vi "nanocal -- nuclear schottky fit V5.vi"() -> ()   [LabVIEW 2020] (continued)
                n371 = Or(x=w756, y=w763) -> (x .or. y?=w767:bool)
              }
              n372 = And Array Elements(Boolean array=w753) -> (logical AND=w752:bool)
            }
            n373 = for {
              tunnel: [w785] -> w748 mode=indexing
              tunnel: [w783] -> w746 mode=indexing
              tunnel: [w780] -> w750 mode=indexing
              tunnel: w744 -> [w782] mode=indexing
              tunnel: w740 -> [w781]
              n374 = Unbundle(w782) -> ("event data"=w780:string, "file pattern"=w785:string)
              n375 = local read "X selector"() -> (w779:T1)
              n376 = Look In Map(map=w781, key=w780) -> (value=w784:map{T1, dbl})  [unwired: 1 in, 1 out]
              n377 = Look In Map(map=w784, key=w779) -> (value=w783:dbl)  [unwired: 1 in, 1 out]
            }
            n378 = call "array - sorted inexes.vi"("x"=w746) -> ("index array"=w747:i32[])  [unwired: 9 in, 1 out]
            n379 = for {
              tunnel: w747 -> [w775] mode=indexing
              tunnel: w748 -> [w778]
              tunnel: [w777] -> w749 mode=indexing
              tunnel: w750 -> [w776]
              shift-right: [w771] -> w739
              shift-left: w745 -> [w774]
              i -> [w773]
              n380 = Index Array(array=w778, index=w775) -> (element=w777:string)
              n381 = Index Array(array=w776, index=w775) -> (element=w772:string)
              n382 = Insert Into Map(map in=w774, key=w773, value=w772) -> (map out=w771:map{i32, string})  [unwired: 2 out]
            }
            "constrained filename lookup" <- w739
            n383 = property on="selection :|\\" class="Ring (strict)"("Strings []"=w749) -> ()  [unwired: 2 in, 2 out]
          }
          frame "action: constrained filenames select" {
            n384 = local read "constrained filename lookup"() -> (w788:map{i32, string})
            n385 = local read "selection :|\\"() -> (w789:u16)
            n386 = local read "all full filenames"() -> (w790:map{string, path})
            n387 = Look In Map(map=w788, key=w789) -> (value=w791:string)  [unwired: 1 in, 1 out]
            n388 = Look In Map(map=w790, key=w791) -> (value=w792:path)  [unwired: 1 in, 1 out]
            n389 = for {
              N: 1 -> [_]
              tunnel: w786 -> [w794]
              tunnel: w792 -> [w793]
              n390 = local write "Read from file"(w793) -> ()
              n391 = Generate User Event(user event=w794, event data cluster="action: read from file" ("event data")) -> ()  [unwired: 2 in, 2 out]
            }
          }
          frame "action: write mathematica string" {
            n392 = local read "mathematica thing"() -> (w800:map{string, map{T1, dbl}})
            n393 = local read "folder"() -> (w799:path)
            n394 = Build Path(base path=w799, name or relative path="temporarystring.txt") -> (appended path=w798:path)
            n395 = call "string parse mathematica list assosiated array -- V2.vi"("action"=3-lorentzian-heat-response_action."create string" ("derivative"), "Map IN"=w800) -> ("string out"=w796:string)  [unwired: 8 in, 1 out]
            "string OUT" <- w796
            n396 = Write to Text File(file (use dialog)=w798, text=w796) -> ()  [unwired: 2 in, 3 out]
          }
          frame "action: replot colors" {
            # "all -- including kappa0"
            n397 = local read "new selector names"() -> (w811:map{T1, map{T10, string}})
            n398 = local read "state of all selectors"() -> (w829:map{T1, map{bool, dbl}})
            n399 = local read "mathematica thing"() -> (w834:map{string, map{T1, dbl}})
            n400 = local read "X selector"() -> (w804:T1)
            n401 = case shown="\"B (T)\"" w804 {
              tunnel: ["B (T)" "T (K)"] -> w803
              frame "B (T)" {
              }
              frame "T (K)", Default {
              }
            }
            n402 = Look In Map(map=w811, key=w804) -> (value=w810:map{T10, string})  [unwired: 1 in, 1 out]
            n403 = control-ref of="Plot:  colors"() -> (w806:refnum<vi>)
            n404 = Array Subset(array=w833, index=0, length=6 ("index")) -> (w831:T1[])
            n405 = local read "state of all selectors string"() -> (w802:string)
            n406 = Look In Map(map=w810, key=nameformattingitem."nameL") -> (value=w808:string)  [unwired: 1 in, 1 out]
            n407 = call "replace plot - plot ref - V2.vi"("Plot ref in"=w806, "text"=w803, "cursor action"=cursor_action."set Xlabel") -> ("Plot ref out"=w805:refnum<vi>)  [unwired: 13 in, 3 out]
            n408 = Concatenate Strings(w802, w808) -> (w828:string)
            n409 = for {
              tunnel: w834 -> [w873]
              tunnel: w804 -> [w868]
              tunnel: w831 -> [w856] mode=indexing
              tunnel: w829 -> [w869]
              tunnel: w811 -> [w860]
              shift-right: [w864] -> w820
              shift-left: w828 -> [w867]
              tunnel: w802 -> [w865]
              tunnel: [w861] -> w822 mode=indexing
              tunnel: w805 -> [w853]
              n410 = for {
                tunnel: w873 -> [w900] mode=indexing
                tunnel: w856 -> [w899]
                tunnel: [w898] -> w872 mode=indexing if=w892
                tunnel: [w897] -> w871 mode=indexing if=w892
                tunnel: w868 -> [w896]
                tunnel: w869 -> [w895]
                n411 = Unbundle(w900) -> ("Map"=w894:map{T1, dbl})  [unwired: 1 out]
                n412 = for {
                  tunnel: w895 -> [w909] mode=indexing
                  tunnel: w894 -> [w908]
                  tunnel: [w906] -> w893 mode=indexing
                  n413 = Unbundle(w909) -> ("Plost: sweep window"=w907:T1, "map"=w905:map{bool, dbl})
                  n414 = for {
                    tunnel: w905 -> [w912] mode=indexing
                    tunnel: [w911] -> w902
                    tunnel: [w910] -> w903
                    n415 = Unbundle(w912) -> ("ignore side !"=w911:bool, "number OUT"=w910:dbl)
                  }
                  n416 = Look In Map(map=w908, key=w907) -> (value=w904:dbl)  [unwired: 1 in, 1 out]
                  n417 = Equal?(x=w904, y=w903) -> (x = y?=w901:bool)
                  n418 = Or(x=w902, y=w901) -> (x .or. y?=w906:bool)
                }
                n419 = Look In Map(map=w894, key=w896) -> (value=w898:dbl)  [unwired: 1 in, 1 out]
                n420 = Look In Map(map=w894, key=w899) -> (value=w897:dbl)  [unwired: 1 in, 1 out]
                n421 = And Array Elements(Boolean array=w893) -> (logical AND=w892:bool)
              }
              n422 = Look In Map(map=w860, key=w856) -> (value=w858:map{T10, string})  [unwired: 1 in, 1 out]
              n423 = Look In Map(map=w858, key=nameformattingitem."nameL") -> (value=w857:string)  [unwired: 1 in, 1 out]
              n424 = call <vilib>:"Space Constant.vi"() -> ("String"=w866:string)
              n425 = Concatenate Strings(w867, w866, w865, w857) -> (w864:string)
              n426 = local read "cursor index map"() -> (w854:map{T1, i32})
              n427 = call "array - sorted inexes.vi"("x"=w872) -> ("index array"=w870:i32[])  [unwired: 9 in, 1 out]
              n428 = local read "color Map"() -> (w855:map{T1, u32})
              n429 = for {
                tunnel: w872 -> [w891]
                tunnel: w871 -> [w890]
                tunnel: w870 -> [w887] mode=indexing
                tunnel: [w889] -> w863 mode=indexing
                tunnel: [w888] -> w862 mode=indexing
                n430 = Index Array(array=w891, index=w887) -> (element=w889:dbl)
                n431 = Index Array(array=w890, index=w887) -> (element=w888:dbl)
              }
              n432 = case shown="\"ζ\"..\"τC\", Default" w856 {
                selector: w856 -> [_ w882]
                tunnel: w863 -> [_ w884]
                tunnel: w862 -> [_ w883]
                tunnel: w855 -> [_ w881]
                tunnel: w854 -> [_ w880]
                tunnel: w853 -> [_ w879]
                frame "κ0" {
                }
                frame "ζ".."τC", Default {
                  n433 = Look In Map(map=w880, key=w882) -> (value=w875:i32)  [unwired: 1 in, 1 out]
                  n434 = call "replace plot - plot ref - V2.vi"("Plot ref in"=w879, "Array X IN"=w884, "Array Y IN"=w883, "plot index"=w875, "cursor action"=cursor_action."write") -> ("Plot ref out"=w878:refnum<vi>)  [unwired: 11 in, 3 out]
                  n435 = Look In Map(map=w881, key=w882) -> (value=w874:u32)  [unwired: 1 in, 1 out]
                  n436 = call "replace cursor - plot ref - V2.vi"("Plot ref in"=w878, "cursor index"=w875, "cursor action"=cursor_action."set cursor color", "Color Box"=w874) -> ("Plot ref out"=w877:refnum<vi>)  [unwired: 12 in, 3 out]
                  n437 = call "replace plot - plot ref - V2.vi"("Plot ref in"=w877, "plot index"=w875, "cursor action"=cursor_action."set plot color", "Color Box"=w874) -> ()  [unwired: 12 in, 4 out]
                }
              }
              n438 = Bundle(w863, w862) -> (w861:cluster{dbl[], dbl[]})  [unwired: 1 in]
            }
            n439 = Index Array(array=w822, index=0) -> (element=w826:cluster{dbl[], dbl[]})
            n440 = local read "folder"() -> (w817:path)
            n441 = Unbundle(w826) -> (w825:dbl[])  [unwired: 1 out]
            n442 = Concatenate Strings("plotstring", w802, ".dat") -> (w812:string)
            n443 = Concatenate Strings(w820, "\r") -> (w818:string)
            n444 = Build Array(w825) -> (w824:dbl[][])
            n445 = for {
              shift-right: [w850] -> w823
              shift-left: w824 -> [w852]
              tunnel: w822 -> [w849] mode=indexing
              n446 = Unbundle(w849) -> (w851:dbl[])  [unwired: 1 out]
              n447 = Build Array (concatenate)(w852, w851) -> (w850:dbl[][])
            }
            n448 = Build Path(base path=w817, name or relative path=w812) -> (appended path=w816:path)
            n449 = Transpose 2D Array(2D array=w823) -> (transposed array=w821:dbl[][])
            n450 = for {
              shift-right: [w842] -> w815
              shift-left: w818 -> [w841]
              tunnel: w821 -> [w839] mode=indexing
              n451 = for {
                shift-right: [w843] -> w838
                shift-left: "" -> [w848]
                tunnel: w839 -> [w847] mode=indexing
                n452 = Number To Fractional String(number=w847, precision (6)=i16 16) -> (F-format string=w845:string)  [unwired: 2 in]
                n453 = Concatenate Strings(w848, w845, "    ") -> (w843:string)
              }
              n454 = Concatenate Strings(w841, w838, "\r") -> (w842:string)
            }
            n455 = Write to Text File(file (use dialog)=w816, text=w815) -> ()  [unwired: 2 in, 3 out]
          }
          frame "action: update state of selectors" {
            w932 = T1[] [enum."T (K)", enum."B (T)", enum."θ (deg)", enum."side (S|R)"] items=["ζ", "τ1", "τS", "τN", "τC", "κ0", "m1", "m2", "m3", "T (K)", "B (T)", "θ (deg)", "side (S|R)", "set of (B|T)", "Re(offset)", "Im(offset)"]
            n456 = local read "selector"() -> (w928:T12)
            n457 = local read "new selector names"() -> (w935:map{T1, map{T10, string}})
            n458 = Unbundle By Name(w928) -> ("side (8S|4R)"=w927:i32, "ignore side !"=w926:bool, "lookup.side lookup"=w925:map{i32, dbl}, "T (K)"=w922:u16, "ignore T !"=w924:bool, "lookup.T lookup"=w923:map{i32, dbl}, "B (T)"=w919:u16, "ignore B !"=w921:bool, "lookup.B lookup"=w920:map{i32, dbl}, "θ (deg)"=w917:u16, "ignore θ !"=w916:bool, "lookup.θ lookup"=w918:map{i32, dbl}, "set (1T|2B)"=w913:i32, "ignore set of !"=w914:bool, "lookup.set of lookup"=w915:map{i32, dbl})
            n459 = Generate User Event(user event=w937, event data cluster="action: replot colors" ("event data")) -> (user event out=w938:refnum<user-event>)  [unwired: 2 in, 1 out]
            n460 = Generate User Event(user event=w938, event data cluster="action: update constrained file selector" ("event data")) -> ()  [unwired: 2 in, 2 out]
            n461 = Look In Map(map=w925, key=w927) -> (value=w931:dbl)  [unwired: 1 in, 1 out]
            n462 = node(w926, w931) -> (w953:map{bool, dbl})
            n463 = Look In Map(map=w923, key=w922) -> (value=w952:dbl)  [unwired: 1 in, 1 out]
            n464 = Look In Map(map=w920, key=w919) -> (value=w948:dbl)  [unwired: 1 in, 1 out]
            n465 = node(w924, w952) -> (w950:map{bool, dbl})
            n466 = node(w921, w948) -> (w947:map{bool, dbl})
            n467 = Look In Map(map=w918, key=w917) -> (value=w946:dbl)  [unwired: 1 in, 1 out]
            n468 = node(w916, w946) -> (w944:map{bool, dbl})
            n469 = Look In Map(map=w915, key=w913) -> (value=w943:dbl)  [unwired: 1 in, 1 out]
            n470 = node(w914, w943) -> (w941:map{bool, dbl})
            n471 = local read "side map from NUM"() -> (w929:map{i32, T8})
            n472 = node(3-lorentzian-parameters."side (S|R)" ("Plost: sweep window"), w953, 3-lorentzian-parameters."T (K)" ("Plost: sweep window"), w950, 3-lorentzian-parameters."B (T)" ("Plost: sweep window"), w947, 3-lorentzian-parameters."θ (deg)" ("Plost: sweep window"), w944, 3-lorentzian-parameters."set of (B|T)" ("Plost: sweep window"), w941) -> (w936:map{T1, map{bool, dbl}})
            "state of all selectors" <- w936
            n473 = for {
              shift-right: [w961] -> _
              shift-left: w936 -> [w961]
              tunnel: w935 -> [w957]
              shift-right: [w960] -> w933
              shift-left: "_" ("event data") -> [w959]
              tunnel: w932 -> [w956] mode=indexing
              n474 = Look In Map(map=w957, key=w956) -> (value=w955:map{T10, string})  [unwired: 1 in, 1 out]
              n475 = Look In Map(map=w961, key=w956) -> (value=w963:map{bool, dbl})  [unwired: 1 in, 1 out]
              n476 = for {
                tunnel: w963 -> [w978] mode=indexing
                tunnel: [w977] -> w962
                tunnel: [w976] -> w958
                n477 = Unbundle(w978) -> ("ignore side ! 2"=w977:bool, "number OUT"=w976:dbl)
              }
              n478 = case shown="False" w962 {
                tunnel: [w974 w975] -> w960
                tunnel: w959 -> [w973 w975]
                tunnel: w958 -> [w970 _]
                tunnel: w955 -> [w966 _]
                frame False {
                  n479 = Look In Map(map=w966, key=nameformattingitem."prec") -> (value=w964:string)  [unwired: 1 in, 1 out]
                  n480 = Look In Map(map=w966, key=nameformattingitem."units") -> (value=w967:string)  [unwired: 1 in, 1 out]
                  n481 = Format Value(format string=w964, value (0)=w970) -> (output string=w969:string)  [unwired: 1 in]
                  n482 = Concatenate Strings(w973, "_" ("event data"), w969, w967, "_" ("event data")) -> (w974:string)
                }
                frame True {
                }
              }
            }
            "state of all selectors string" <- w933
            n483 = Look In Map(map=w929, key=w931) -> (value=w930:T8)  [unwired: 1 in, 1 out]
            n484 = local write "side"(w930) -> ()
          }
          frame "action: reset colors" {
            w985 = map{T1, u32} {}  # Size: 0
            n485 = local read "parameter"() -> (w992:T1[])
            n486 = local read "colors"() -> (w994:u32[])
            n487 = for {
              shift-right: [w997] -> w993
              shift-left: w985 -> [w998]
              tunnel: w992 -> [w996] mode=indexing
              tunnel: w994 -> [w995] mode=indexing
              n488 = Insert Into Map(map in=w998, key=w996, value=w995) -> (map out=w997:map{T1, u32})  [unwired: 2 out]
            }
            n489 = local write "color Map"(w993) -> ()
            n490 = Look In Map(map=w993, key=3-lorentzian-parameters."ζ" ("Plost: sweep window")) -> (value=w991:u32)  [unwired: 1 in, 1 out]
            n491 = Look In Map(map=w993, key=3-lorentzian-parameters."τ1" ("Plost: sweep window")) -> (value=w990:u32)  [unwired: 1 in, 1 out]
            n492 = Look In Map(map=w993, key=3-lorentzian-parameters."τS" ("Plost: sweep window")) -> (value=w989:u32)  [unwired: 1 in, 1 out]
            n493 = Look In Map(map=w993, key=3-lorentzian-parameters."τN" ("Plost: sweep window")) -> (value=w988:u32)  [unwired: 1 in, 1 out]
            n494 = Look In Map(map=w993, key=3-lorentzian-parameters."τC" ("Plost: sweep window")) -> (value=w987:u32)  [unwired: 1 in, 1 out]
            n495 = Look In Map(map=w993, key=3-lorentzian-parameters."κ0" ("Plost: sweep window")) -> (value=w986:u32)  [unwired: 1 in, 1 out]
            n496 = property on="ζ" class="Slide (strict)"("Fill Color"=w991) -> ()  [unwired: 2 in, 2 out]
            n497 = property on="T1" class="Slide (strict)"("Fill Color"=w990) -> ()  [unwired: 2 in, 2 out]
            n498 = property on="τS" class="Slide (strict)"("Fill Color"=w989) -> ()  [unwired: 2 in, 2 out]
            n499 = property on="τN" class="Slide (strict)"("Fill Color"=w988) -> ()  [unwired: 2 in, 2 out]
            n500 = property on="τC" class="Slide (strict)"("Fill Color"=w987) -> ()  [unwired: 2 in, 2 out]
            n501 = property on="κ0" class="Slide (strict)"("Fill Color"=w986) -> ()  [unwired: 2 in, 2 out]
          }
          frame "action: copy from math" {
            w1007 = map{T1, bool} {}  # Size: 0
            n502 = local read "default selector"() -> (w1006:T11)
            n503 = case shown="True" "overwrite offset" {
              tunnel: w1004 -> [w1017 w1021]
              tunnel: [w1017 w1020] -> w1003
              frame False {
              }
              frame True {
                n504 = Build Array (concatenate)(w1021, 3-lorentzian-parameters."Re(offset)" ("Plost: sweep window"), 3-lorentzian-parameters."Im(offset)" ("Plost: sweep window")) -> (w1020:T1[])
              }
            }
            n505 = local read "mathematica thing"() -> (w1012:map{string, map{T1, dbl}})
            n506 = for {
              shift-right: [w1025] -> w1005
              shift-left: w1007 -> [w1026]
              tunnel: w1006 -> [w1024] mode=indexing
              n507 = Unbundle(w1024) -> ("Plost: sweep window"=w1023:T1, "used default"=w1022:bool)
              n508 = Insert Into Map(map in=w1026, key=w1023, value=w1022) -> (map out=w1025:map{T1, bool})  [unwired: 2 out]
            }
            n509 = local read "key"() -> (w1011:string)
            n510 = Look In Map(map=w1012, key=w1011) -> (key not found?=w1009:bool, value=w1010:map{T1, dbl})  [unwired: 1 in]
            n511 = case shown="False" w1009 {
              tunnel: w1010 -> [w1048 _]
              tunnel: w1005 -> [w1046 _]
              tunnel: w1003 -> [w1047 _]
              tunnel: "overwrite offset" -> [w1028 w1076]
              tunnel: [w1027 w1076] -> w1001
              frame False {
                # "the order of numbers \nMUST corrspond to order\nin the \"parameter\" array"
                n512 = for {
                  tunnel: [w1056] -> w1045 mode=indexing
                  tunnel: w1048 -> [w1060]
                  tunnel: w1047 -> [w1054] mode=indexing
                  tunnel: w1046 -> [w1059]
                  n513 = Look In Map(map=w1059, key=w1054, default value=FALSE) -> (value=w1058:bool)  [unwired: 1 out]
                  n514 = Look In Map(map=w1060, key=w1054) -> (value=w1057:dbl)  [unwired: 1 in, 1 out]
                  n515 = case shown="True" w1058 {
                    tunnel: w1057 -> [w1061 _]
                    tunnel: w1054 -> [_ w1074]
                    tunnel: [w1061 w1062] -> w1056
                    tunnel: w1054 -> [_ w1072]
                    frame False {
                    }
                    frame True {
                      n516 = local read "B (T)"() -> (w1069:dbl)
                      n517 = local read "T (K)"() -> (w1075:dbl)
                      n518 = Divide(x=w1069, y=12.0) -> (x/y=w1067:dbl)
                      n519 = Square(x=w1067) -> (x^2=w1066:dbl)
                      n520 = Equal?(x=3-lorentzian-parameters."τN", y=w1072) -> (x = y?=w1070:bool)
                      n521 = call "nanocal -- defaut parameter manager -- V1.vi"("action"=nanocal_--_defaut_parameter_manager_action--_V1."get logarithmic interp", "T"=w1075, "what"=w1074) -> ("number"=w1064:dbl)  [unwired: 8 in]
                      n522 = Select(t=w1066, s=w1070, f=1.0) -> (s? t:f=w1063:dbl)
                      n523 = Multiply(x=w1064, y=w1063) -> (x*y=w1062:dbl)
                    }
                  }
                }
                n524 = Index Array(array=w1045, index #1=0 ("index"), index #2=1 ("index"), index #3=2 ("index"), index #4=3 ("index"), index #5=4 ("index"), index #6=5 ("index"), index #7=6 ("index"), index #8=7 ("index")) -> (element #1=w1042:dbl, element #2=w1041:dbl, element #3=w1036:dbl, element #4=w1035:dbl, element #5=w1034:dbl, element #6=w1033:dbl, element #7=w1030:dbl, element #8=w1029:dbl)
                n525 = case shown="False" w1028 {
                  selector: w1028 -> [w1049 w1050]
                  tunnel: w1030 -> [_ w1052]
                  tunnel: w1029 -> [_ w1051]
                  tunnel: [w1049 w1050] -> w1027
                  frame False {
                  }
                  frame True {
                    n526 = Bundle("number"=w1052, "number"=w1051) -> (w1053:cluster{"number":dbl, "number":dbl})  [unwired: 1 in]
                    n527 = local write "offset Re\noffset Im"(w1053) -> ()
                  }
                }
                n528 = local write "ζ"(w1042) -> ()
                n529 = local write "T1"(w1041) -> ()
                n530 = local write "τS"(w1036) -> ()
                n531 = local write "τN"(w1035) -> ()
                n532 = local write "τC"(w1034) -> ()
                n533 = local write "κ0"(w1033) -> ()
              }
              frame True {
              }
            }
            n534 = case shown="True" w1001 {
              tunnel: w1008 -> [w1013 w1015]
              tunnel: [w1013 w1014] -> w999
              frame False {
              }
              frame True {
                n535 = Generate User Event(user event=w1015, event data cluster="action: read from file" ("event data")) -> (user event out=w1014:refnum<user-event>)  [unwired: 2 in, 1 out]
              }
            }
            n536 = Generate User Event(user event=w999, event data cluster="action: new sweep" ("event data")) -> ()  [unwired: 2 in, 2 out]
          }
          frame "action: copy to math" {
            w1090 = 0.0
            w1085 = T1[] [enum."ζ", enum."τ1", enum."τS", enum."τN", enum."τC", enum."κ0", enum."m1", enum."m2", enum."m3", enum."T (K)", enum."B (T)", enum."θ (deg)", enum."Re(offset)", enum."Im(offset)"] items=["ζ", "τ1", "τS", "τN", "τC", "κ0", "m1", "m2", "m3", "T (K)", "B (T)", "θ (deg)", "side (S|R)", "set of (B|T)", "Re(offset)", "Im(offset)"]
            n537 = local read "offset Re\noffset Im"() -> (w1079:cluster{"Numeric":dbl, "Numeric":dbl})
            n538 = local read "θ (deg)"() -> (w1087:dbl)
            n539 = local read "T (K)"() -> (w1089:dbl)
            n540 = local read "B (T)"() -> (w1088:dbl)
            n541 = Unbundle(w1079) -> ("Numeric"=w1078:dbl, "Numeric"=w1077:dbl)
            n542 = local read "τN"() -> (w1096:dbl)
            n543 = local read "τC"() -> (w1095:dbl)
            n544 = local read "T1"() -> (w1098:dbl)
            n545 = local read "κ0"() -> (w1094:dbl)
            n546 = local read "τS"() -> (w1097:dbl)
            n547 = local read "ζ"() -> (w1099:dbl)
            n548 = Build Array(w1099, w1098, w1097, w1096, w1095, w1094, w1090, w1090, w1090, w1089, w1088, w1087, w1078, w1077) -> (w1086:dbl[])
            n549 = Generate User Event(user event=w1100, event data cluster="action: replot colors" ("event data")) -> ()  [unwired: 2 in, 2 out]
            n550 = for {
              tunnel: w1086 -> [w1102] mode=indexing
              tunnel: w1085 -> [w1103] mode=indexing
              tunnel: [w1103] -> w1084 mode=indexing
              shift-right: [w1104] -> w1082
              shift-left: map{T1, dbl} {} ("Map") -> [w1105]
              n551 = Insert Into Map(map in=w1105, key=w1103, value=w1102) -> (map out=w1104:map{T1, dbl})  [unwired: 2 out]
            }
            n552 = local read "mathematica thing"() -> (w1093:map{string, map{T1, dbl}})
            n553 = local read "key"() -> (w1092:string)
            n554 = call "3-lorentzian-heat-response -- V4.vi"("action"=3-lorentzian-heat-response_action."calc m1m2m3", "Map IN"=w1082) -> ("Map OUT"=w1081:map{T1, dbl})  [unwired: 7 in, 2 out]
            n555 = in-place {
              in-place-border: w1084 -> [w1110]
              in-place-border: w1081 -> [w1106]
              n556 = in-place-map #4(w1093, w1092) -> (w1109:map{T1, dbl})  [unwired: 1 in, 1 out]
              n557 = for {
                tunnel: w1110 -> [w1112] mode=indexing
                shift-right: [w1114] -> w1108
                shift-left: w1109 -> [w1115]
                shift-right: [w1113] -> _
                shift-left: w1106 -> [w1113]
                n558 = Look In Map(map=w1113, key=w1112) -> (value=w1111:dbl)  [unwired: 1 in, 1 out]
                n559 = Insert Into Map(map in=w1115, key=w1112, value=w1111) -> (map out=w1114:map{T1, dbl})  [unwired: 2 out]
              }
              n560 = in-place-map #4(w1108, LVMapReplaceAction."Modify Entry only if found" ("action")) -> (w1091:map{string, map{T1, dbl}})  [unwired: 2 out]
            }
            n561 = local write "mathematica thing"(w1091) -> ()
          }
          frame "action: exit" {
          }
          frame "action: read from file" {
            n562 = local read "Read from file"() -> (w1117:path)
            n563 = Unbundle("offset Re\noffset Im") -> ("Numeric"=w1142:dbl, "Numeric"=w1141:dbl)
            n564 = Re/Im To Complex(1:w1141, 2:w1142) -> (0:w1129:cdb)
            n565 = call "file - read-write - list of lines-V2.vi"("read/write control"=file_--_read-write_control."read", "file path"=w1117) -> ("header OUT"=w1126:string, "list of lines OUT"=w1128:string[], "filename out"=w1156:string)  [unwired: 7 in]
            n566 = Generate User Event(user event=w1157, event data cluster="action: new sweep" ("event data")) -> ()  [unwired: 2 in, 2 out]
            n567 = local read "cursor x selector"() -> (w1139:map{T1, dbl})
            n568 = call "filename-manage.vi"("filename-action"=filename-action."get name", "file name IN"=w1156) -> ("string OUT"=w1125:string)  [unwired: 7 in, 2 out]
            n569 = call "filename-manage.vi"("filename-action"=filename-action."get T", "file name IN"=w1125) -> ("number OUT"=w1138:dbl, "filename OUT"=w1153:string)  [unwired: 7 in, 1 out]
            "T (K)" <- w1138
            n570 = case shown="\"raw nanocal\"" "data file formatting" {
              tunnel: [w1162 w1180 w1216 w1243] -> w1150
              tunnel: [w1161 w1179 w1215 w1242] -> w1144
              tunnel: w1129 -> [w1160 w1182 w1211 w1232]
              tunnel: w1128 -> [w1163 w1190 w1210 w1231]
              tunnel: w1126 -> [_ w1191 _ _]
              tunnel: w1125 -> [_ w1177 _ _]
              tunnel: w1117 -> [_ w1181 _ _]
              tunnel: "side" -> [_ w1176 _ _]
              frame "as is", Default {
                n571 = for {
                  tunnel: w1163 -> [w1174] mode=indexing
                  tunnel: [w1169] -> w1164 mode=indexing if=w1165
                  tunnel: [w1168] -> w1162 mode=indexing if=w1165
                  w1170 = 0.0
                  n572 = Scan From String(format string="%f%f%f", input string=w1174, initial scan location=u32 0, default 1=w1170, default 2=w1170, default 3=w1170) -> (offset past scan=w1166:u32, output 1=w1168:dbl, output 2=w1172:dbl, output 3=w1171:dbl)  [unwired: 1 in, 2 out]
                  n573 = Greater Than 0?(x=w1166) -> (x > 0?=w1165:bool)
                  n574 = Re/Im To Complex(1:w1171, 2:w1172) -> (0:w1169:cdb)
                }
                n575 = Subtract(x=w1164, y=w1160) -> (x-y=w1161:cdb[])
              }
              frame "raw nanocal" {
                n576 = case shown="\"ref\"" w1176 {
                  tunnel: [nanocal_raw_file_manage_action_V1."read S side" ("action") nanocal_raw_file_manage_action_V1."read R side" ("action")] -> w1175
                  frame "sam", Default {
                  }
                  frame "ref" {
                  }
                }
                n577 = call "nanocal_raw_file_manage_V1.vi"("action"=w1175, "list of lines IN"=w1190, "header IN"=w1191) -> ("z (K/W)  OUT"=w1183:cdb[], "f (Hz) OUT"=w1184:dbl[])  [unwired: 6 in, 1 out]
                n578 = Subtract(x=w1183, y=w1182) -> (x-y=w1185:cdb[])
                n579 = call "array -- freq-voltage transformations.vi"("freq voltage action"=array_--_freq-voltage_transformations_action."add -ω", "z In"=w1185, "ω IN"=w1184) -> ("z out"=w1188:cdb[], "ω out"=w1189:dbl[])  [unwired: 5 in, 2 out]
                n580 = call "array -- freq-voltage transformations.vi"("freq voltage action"=array_--_freq-voltage_transformations_action."sort ω", "z In"=w1188, "ω IN"=w1189) -> ("z out"=w1179:cdb[], "ω out"=w1180:dbl[])  [unwired: 5 in, 2 out]
                n581 = case shown="True" "toggle generate labview files" {
                  tunnel: w1181 -> [_ w1203]
                  tunnel: w1177 -> [_ w1207]
                  tunnel: w1180 -> [_ w1199]
                  tunnel: w1179 -> [_ w1198]
                  frame False {
                  }
                  frame True {
                    n582 = call "filename-manage.vi"("filename-action"=filename-action."get basename", "file name IN"=w1207) -> ("string OUT"=w1205:string)  [unwired: 7 in, 2 out]
                    n583 = Concatenate Strings(w1205, "_labview_.dat") -> (w1194:string)
                    n584 = Strip Path(path=w1203) -> (stripped path=w1202:path)  [unwired: 1 out]
                    n585 = call "array -- freq-voltage transformations.vi"("freq voltage action"=array_--_freq-voltage_transformations_action."labview file str", "z In"=w1198, "ω IN"=w1199) -> ("lines out"=w1196:string[], "header OUT"=w1197:string)  [unwired: 5 in, 2 out]
                    n586 = Build Path(base path=w1202, name or relative path=w1194) -> (appended path=w1201:path)
                    n587 = call "file - read-write - list of lines-V2.vi"("read/write control"=file_--_read-write_control."write all", "header IN"=w1197, "list of lines IN"=w1196, "file path"=w1201) -> ()  [unwired: 5 in, 3 out]
                  }
                }
              }
              frame "add - ω" {
                n588 = for {
                  tunnel: w1210 -> [w1228] mode=indexing
                  tunnel: [w1223] -> w1212 mode=indexing if=w1219
                  tunnel: [w1222] -> w1208 mode=indexing if=w1219
                  w1224 = 0.0
                  n589 = Scan From String(format string="%f%f%f", input string=w1228, initial scan location=u32 0, default 1=w1224, default 2=w1224, default 3=w1224) -> (offset past scan=w1220:u32, output 1=w1222:dbl, output 2=w1226:dbl, output 3=w1225:dbl)  [unwired: 1 in, 2 out]
                  n590 = Greater Than 0?(x=w1220) -> (x > 0?=w1219:bool)
                  n591 = Re/Im To Complex(1:w1225, 2:w1226) -> (0:w1223:cdb)
                }
                n592 = Subtract(x=w1212, y=w1211) -> (x-y=w1209:cdb[])
                n593 = call "array -- freq-voltage transformations.vi"("freq voltage action"=array_--_freq-voltage_transformations_action."add -ω", "z In"=w1209, "ω IN"=w1208) -> ("z out"=w1217:cdb[], "ω out"=w1218:dbl[])  [unwired: 5 in, 2 out]
                n594 = call "array -- freq-voltage transformations.vi"("freq voltage action"=array_--_freq-voltage_transformations_action."sort ω", "z In"=w1217, "ω IN"=w1218) -> ("z out"=w1215:cdb[], "ω out"=w1216:dbl[])  [unwired: 5 in, 2 out]
              }
              frame "full rydh" {
                n595 = for {
                  tunnel: w1231 -> [w1255] mode=indexing
                  tunnel: [w1250] -> w1233 mode=indexing if=w1246
                  tunnel: [w1249] -> w1229 mode=indexing if=w1246
                  w1251 = 0.0
                  n596 = Scan From String(format string="%f%f%f", input string=w1255, initial scan location=u32 0, default 1=w1251, default 2=w1251, default 3=w1251) -> (offset past scan=w1247:u32, output 1=w1249:dbl, output 2=w1253:dbl, output 3=w1252:dbl)  [unwired: 1 in, 2 out]
                  n597 = Greater Than 0?(x=w1247) -> (x > 0?=w1246:bool)
                  n598 = Re/Im To Complex(1:w1252, 2:w1253) -> (0:w1250:cdb)
                }
                n599 = Subtract(x=w1233, y=w1232) -> (x-y=w1230:cdb[])
                n600 = call "array -- freq-voltage transformations.vi"("freq voltage action"=array_--_freq-voltage_transformations_action."2 x ω", "z In"=w1230, "ω IN"=w1229) -> ("z out"=w1237:cdb[], "ω out"=w1239:dbl[])  [unwired: 5 in, 2 out]
                n601 = call "array -- freq-voltage transformations.vi"("freq voltage action"=array_--_freq-voltage_transformations_action."R-phase(deg) to Re-Im", "z In"=w1237, "ω IN"=w1239) -> ("z out"=w1236:cdb[], "ω out"=w1238:dbl[])  [unwired: 5 in, 2 out]
                n602 = call "array -- freq-voltage transformations.vi"("freq voltage action"=array_--_freq-voltage_transformations_action."add -ω", "z In"=w1236, "ω IN"=w1238) -> ("z out"=w1244:cdb[], "ω out"=w1245:dbl[])  [unwired: 5 in, 2 out]
                n603 = call "array -- freq-voltage transformations.vi"("freq voltage action"=array_--_freq-voltage_transformations_action."sort ω", "z In"=w1244, "ω IN"=w1245) -> ("z out"=w1242:cdb[], "ω out"=w1243:dbl[])  [unwired: 5 in, 2 out]
              }
            }
            n604 = Insert Into Map(map in=w1139, key=3-lorentzian-parameters."T (K)" ("Plost: sweep window"), value=w1138) -> (map out=w1137:map{T1, dbl})  [unwired: 2 out]
            n605 = call "filename-manage.vi"("filename-action"=filename-action."get deg", "file name IN"=w1153) -> ("number OUT"=w1134:dbl, "filename OUT"=w1120:string)  [unwired: 7 in, 1 out]
            "θ (deg)" <- w1134
            n606 = Insert Into Map(map in=w1137, key=3-lorentzian-parameters."θ (deg)" ("Plost: sweep window"), value=w1134) -> (map out=w1136:map{T1, dbl})  [unwired: 2 out]
            n607 = local read "side map to STR"() -> (w1118:map{T8, string})
            n608 = call "filename-manage.vi"("filename-action"=filename-action."get B", "file name IN"=w1120) -> ("number OUT"=w1133:dbl, "filename OUT"=w1119:string)  [unwired: 7 in, 1 out]
            "B (T)" <- w1133
            n609 = call "filename-manage.vi"("filename-action"=filename-action."getIDStock", "file name IN"=w1119) -> ("string OUT"=w1123:string)  [unwired: 7 in, 2 out]
            "file IDS" <- w1123
            n610 = Look In Map(map=w1118, key="side") -> (value=w1124:string)  [unwired: 1 in, 1 out]
            n611 = Insert Into Map(map in=w1136, key=3-lorentzian-parameters."B (T)" ("Plost: sweep window"), value=w1133) -> (map out=w1135:map{T1, dbl})  [unwired: 2 out]
            n612 = Concatenate Strings(w1123, w1124) -> (→"key":string)
            n613 = local write "cursor x selector"(w1135) -> ()
            n614 = call "filter - complex - four.vi"("omega (Hz) in"=w1150, "z in"=w1144, "span"="cspan") -> ("omega out"=w1149:dbl[], "z out"=w1148:cdb[], "dz/domega out"=w1147:cdb[])  [unwired: 9 in, 5 out]
            n615 = call "nanocal -- publish -- freq scan V2.vi"("publisher action"=publisher_action."set", "dz/dω IN (V)"=w1147, "z IN (V)"=w1148, "ω IN (Hz)"=w1149) -> ()  [unwired: 4 in, 4 out]
          }
          frame "action: save freq scan" {
            n616 = local read "Freq sweep name template"() -> (w1261:T7)
            n617 = call "MFLI -- publish -- freq scan.vi"("publisher action"=publisher_action."get") -> ("Voltage out (V)"=w1257:cdb[], "Freq out (Hz)"=w1258:dbl[])  [unwired: 9 in]
            n618 = call "filename-manage.vi"("filename pattern"=w1261, "filename-action"=filename-action."uniquenum", "folder IN"="Save folder", "file name IN"="freq sweep file name") -> ("filename OUT"=w1260:string)  [unwired: 5 in, 2 out]
            n619 = call "KM_appendline -- freq sweep.vi"("freq"=w1258, "Vout(V)"=w1257, "Save frequency scan"="Save folder", "read/write control"=KM_file_--_read-write_control."append one line", "name or relative path"=w1260) -> ()  [unwired: 15 in]
            n620 = local write "freq sweep file name"(w1260) -> ()
          }
          frame "void", Default {
          }
        }
      }
    }
  }
  n621 = while "interface" {
    tunnel: w34 -> [w1269]
    tunnel: w23 -> [w1268]
    tunnel: w20 -> [w1266]
    tunnel: w17 -> [w1265]
    tunnel: w16 -> [_]
    stop <- w1267 stop-if-true
    n622 = event shown="[14] \"Plot:  colors\": Cursor Move" {
      selector: w1269 -> [_ _ _ _ _ _ _ _ _ _ _ _ _ _ _ _ _ _ _ _ _ _ _ _ _ _ _ _]
      dyn-events: _ -> [_ _ _ _ _ _ _ _ _ _ _ _ _ _ _ _ _ _ _ _ _ _ _ _ _ _ _ _]
      timeout: _ -> [_ _ _ _ _ _ _ _ _ _ _ _ _ _ _ _ _ _ _ _ _ _ _ _ _ _ _ _]
      tunnel: w1268 -> [w1270 _ w1282 w1284 _ w1313 w1315 w1318 w1323 w1325 w1327 w1329 w1332 w1338 w1420 _ w1448 w1451 w1453 w1457 w1460 w1463 w1466 w1474 w1478 _ w1526 w1529]
      tunnel: [_ _ _ _ _ _ _ _ "load! :l" _ _ _ _ _ _ _ _ _ _ _ _ _ _ _ _ _ _ _] -> _
      tunnel: [_ _ _ _ _ _ _ _ _ _ _ _ _ _ _ _ _ _ _ _ _ _ _ _ _ w1480 _ _] -> w1267
      tunnel: [_ _ _ _ _ "go!" _ _ _ _ _ _ "parse! :p" _ _ "pause!" "uco! :u" "Math→τ! :q" _ "τ→Math! :p" "Math→ string OUT! :s" "generate empty string from filelist !" "string IN → Math!" _ _ _ "plot landscape!" _] -> _
      tunnel: w1266 -> [_ _ _ _ _ _ _ _ _ _ _ _ _ w1334 _ _ _ _ _ _ _ _ _ _ _ _ _ _]
      tunnel: w1265 -> [_ _ _ _ _ _ _ _ _ _ _ _ _ _ w1443 _ _ _ _ _ _ _ _ _ _ _ _ _]
      tunnel: [_ _ _ _ _ _ _ _ _ "Read from file" _ _ _ _ _ _ _ _ _ _ _ _ _ _ _ _ _ _] -> _
      tunnel: [_ _ _ _ _ _ _ _ _ _ _ _ _ _ _ _ _ _ "load default values" _ _ _ _ _ _ _ _ _] -> _
      event "Plot: sweep window": Cursor Move {
        n623 = event-data() -> ("CursIdx"=w1271:i32)  [unwired: 1 in]
        n624 = case shown="0..2" w1271 {
          tunnel: w1270 -> [w1273 _]
          frame 0..2 {
            w1272 = "action: fit"  # action
            n625 = Generate User Event(user event=w1273, event data cluster=w1272) -> ()  [unwired: 2 in, 2 out]
          }
          frame 3..5, Default {
          }
        }
      }
      event "scale gauge: Plot: complex plane": Value Change {
        n626 = event-data() -> ()  [unwired: 1 in, 1 out]
        n627 = local read "scale gauge: Plot: complex plane"() -> (w1280:dbl)
        n628 = control-ref of="Plot: sweep window"() -> (w1279:refnum<vi>)
        n629 = Multiply(x=w1280, y=0.3) -> (x*y=w1281:dbl)
        n630 = Bundle By Name(cluster=T33 {"window y"=0.0021014740628288917, "center x"=44850.89441339177, "center y"=2.5658109925320947, "window x"=17480.201988350764} ("window IN"), "window x"=w1280, "window y"=w1280, "center x"=w1281, "center y"=0.0) -> (w1278:T33)
        n631 = call "replace cursor - plot ref - V2.vi"("Plot ref in"=w1279, "window IN"=w1278, "cursor action"=cursor_action."zoom to win") -> ()  [unwired: 13 in, 4 out]
      }
      event "ζ", "T1", "τS", "τN", "τC", "κ0": Value Change {
        n632 = event-data() -> ()  [unwired: 1 in, 1 out]
        n633 = Generate User Event(user event=w1282, event data cluster="action: new sweep" ("event data")) -> ()  [unwired: 2 in, 2 out]
      }
      event Value Change {
        n634 = event-data() -> ()  [unwired: 1 in, 6 out]
        n635 = Generate User Event(user event=w1284, event data cluster="action: update enums" ("event data")) -> ()  [unwired: 2 in, 2 out]
      }
      event "ω0 (rad/sec)": Value Change {
        n636 = event-data() -> ()  [unwired: 1 in, 1 out]
        n637 = call "nanocal -- publish -- freq scan V2.vi"("publisher action"=publisher_action."get") -> ("z out (V)"=w1311:cdb[], "ω out (Hz)"=w1306:dbl[])  [unwired: 7 in, 2 out]
        n638 = control-ref of="Plot: sweep window"() -> (w1293:refnum<vi>)
        n639 = local read "T1"() -> (w1295:dbl)
        n640 = local read "τN"() -> (w1297:dbl)
        n641 = local read "ζ"() -> (w1294:dbl)
        n642 = local read "τS"() -> (w1296:dbl)
        n643 = local read "τC"() -> (w1298:dbl)
        n644 = local read "κ0"() -> (w1299:dbl)
        n645 = Divide(x="ω0 (rad/sec)", y=6.283185307179586) -> (x/y=w1304:dbl)
        n646 = call "3-lorentzian-heat-response.vi"("zeta"=w1294, "T1"=w1295, "tauS"=w1296, "tauN"=w1297, "tauC"=w1298, "kappa0"=w1299, "omega (rad/sec)"="ω0 (rad/sec)", "action"=3-lorentzian-heat-response_action."calc R") -> ("Romega"=w1302:cdb)  [unwired: 7 in, 4 out]
        n647 = Complex To Re/Im(x + iy=w1302) -> (x=w1300:dbl, y=w1301:dbl)
        n648 = Threshold 1D Array(2:w1304, 3:w1306) -> (0:w1305:dbl)  [unwired: 1 in]
        n649 = call "replace cursor - plot ref - V2.vi"("Plot ref in"=w1293, "new X"=w1300, "new  Y"=w1301, "cursor index"=0, "cursor action"=cursor_action."write") -> ("Plot ref out"=w1307:refnum<vi>)  [unwired: 11 in, 3 out]
        n650 = Index Array(array=w1311, index=w1305) -> (element=w1308:cdb)
        n651 = Complex To Re/Im(x + iy=w1308) -> (x=w1309:dbl, y=w1310:dbl)
        n652 = call "replace cursor - plot ref - V2.vi"("Plot ref in"=w1307, "new X"=w1309, "new  Y"=w1310, "cursor index"=1, "cursor action"=cursor_action."write") -> ()  [unwired: 11 in, 4 out]
      }
      event "go!": Value Change {
        n653 = event-data() -> ()  [unwired: 1 in, 6 out]
        n654 = Generate User Event(user event=w1313, event data cluster="action: gradient step" ("event data")) -> ()  [unwired: 2 in, 2 out]
      }
      event "selector": Value Change {
        n655 = event-data() -> ()  [unwired: 1 in, 6 out]
        n656 = Generate User Event(user event=w1315, event data cluster="action: update state of selectors" ("event data")) -> ()  [unwired: 2 in, 2 out]
      }
      event "Plot: sweep window": Cursor Release {
        n657 = event-data() -> ("CursIdx"=w1317:i32)  [unwired: 1 in]
        n658 = case shown="0..2" w1317 {
          tunnel: w1318 -> [_ w1319]
          frame 3, Default {
          }
          frame 0..2 {
            w1320 = "action: fit"  # event data
            n659 = Generate User Event(user event=w1319, event data cluster=w1320) -> ()  [unwired: 2 in, 2 out]
          }
        }
      }
      event "load! :l": Value Change {
        n660 = event-data() -> ()  [unwired: 1 in, 6 out]
        n661 = Generate User Event "action User Event"(user event=w1323, event data cluster="action: read from file" ("event data")) -> ()  [unwired: 2 in, 2 out]
      }
      event "Read from file": Value Change {
        n662 = event-data() -> ()  [unwired: 1 in, 6 out]
        n663 = Generate User Event "action User Event"(user event=w1325, event data cluster="action: read from file" ("event data")) -> ()  [unwired: 2 in, 2 out]
      }
      event "offset Re\noffset Im": Value Change {
        n664 = event-data() -> ()  [unwired: 1 in, 6 out]
        n665 = Generate User Event "action User Event"(user event=w1327, event data cluster="action: read from file" ("event data")) -> ()  [unwired: 2 in, 2 out]
      }
      event "cspan": Value Change {
        n666 = event-data() -> ()  [unwired: 1 in, 6 out]
        n667 = Generate User Event "action User Event"(user event=w1329, event data cluster="action: read from file" ("event data")) -> ()  [unwired: 2 in, 2 out]
      }
      event "parse! :p": Value Change {
        n668 = event-data() -> ()  [unwired: 1 in, 6 out]
        n669 = Generate User Event "action User Event"(user event=w1332, event data cluster="action: parse string" ("event data")) -> ()  [unwired: 2 in, 2 out]
      }
      event Key Down {
        n670 = event-data() -> ("Char"=w1336:i16, "VKey"=w1339:T34)  [unwired: 1 in]
        n671 = Build Array(w1336) -> (w1337:i16[])
        n672 = Byte Array To String(unsigned byte array=w1337) -> (string=w1335:string)
        n673 = case shown="\"ASCII\", Default" w1339 {
          selector: w1339 -> [_ _ _ _ _ _ w1413]
          tunnel: w1338 -> [w1342 _ _ w1408 _ _ _]
          tunnel: w1335 -> [w1341 _ _ _ _ _ _]
          tunnel: w1334 -> [w1340 _ _ _ _ _ w1412]
          frame "ASCII", Default {
            n674 = case shown="\"<\", \">\"" w1341 {
              selector: w1341 -> [_ _ _ _ _ _ w1356 w1366 _ _ _ _ w1386 _]
              tunnel: w1342 -> [_ _ w1343 w1345 w1348 _ _ _ _ w1377 w1380 w1382 w1384 w1405]
              tunnel: w1340 -> [_ _ _ _ _ w1352 _ _ _ _ _ _ _ _]
              frame "0", Default {
              }
              frame "a" {
              }
              frame "s" {
                n675 = Generate User Event(user event=w1343, event data cluster="action: write mathematica string" ("event data")) -> ()  [unwired: 2 in, 2 out]
              }
              frame "l" {
                n676 = Generate User Event(user event=w1345, event data cluster="action: read from file" ("event data")) -> ()  [unwired: 2 in, 2 out]
              }
              frame " " {
                n677 = Generate User Event(user event=w1348, event data cluster="action: gradient step" ("event data")) -> ()  [unwired: 2 in, 2 out]
              }
              frame "?" {
                # "?"
                n678 = call "replace cursor - plot ref - V2.vi"("Plot ref in"=w1352, "cursor action"=cursor_action."zoom to win") -> ("Plot ref out"=w1351:refnum<vi>)  [unwired: 14 in, 3 out]
                n679 = call "replace cursor - plot ref - V2.vi"("Plot ref in"=w1351, "cursor action"=cursor_action."smart zoom out&aspect") -> ()  [unwired: 14 in, 4 out]
              }
              frame ",", "." {
                n680 = local read "newton parameters"() -> (w1354:T2)
                n681 = case shown="\".\"" w1356 {
                  tunnel: [0.7 1.0 1.5] -> w1355
                  frame "," {
                  }
                  frame "0", Default {
                  }
                  frame "." {
                  }
                }
                n682 = in-place {
                  in-place-border: w1355 -> [w1359]
                  n683 = in-place-cluster #5(w1354) -> ("PID-P"=w1357:dbl)
                  n684 = Multiply(x=w1359, y=w1357) -> (x*y=w1358:dbl)
                  n685 = in-place-cluster #5("PID-P"=w1358) -> (w1353:T2)
                }
                n686 = local write "newton parameters"(w1353) -> ()
              }
              frame "<", ">" {
                n687 = local read "newton parameters"() -> (w1364:T2)
                n688 = case shown="\"<\"" w1366 {
                  tunnel: [-5 0 5] -> w1365
                  frame "<" {
                  }
                  frame "0", Default {
                  }
                  frame ">" {
                  }
                }
                n689 = in-place {
                  in-place-border: w1365 -> [w1372]
                  n690 = in-place-cluster #6(w1364) -> ("PID-I"=w1371:i32)
                  n691 = Add(x=w1372, y=w1371) -> (x+y=w1370:i32)
                  n692 = In Range and Coerce(upper limit=100, x=w1370, lower limit=2) -> (coerced(x)=w1367:i32)  [unwired: 1 out]
                  n693 = in-place-cluster #6("PID-I"=w1367) -> (w1363:T2)
                }
                n694 = local write "newton parameters"(w1363) -> ()
              }
              frame "b" {
                n695 = local read "String"() -> (w1376:string)
                n696 = local write "backup string :b"(w1376) -> ()
              }
              frame "u" {
                n697 = Generate User Event(user event=w1377, event data cluster="ignoreaction: uco" ("event data")) -> ()  [unwired: 2 in, 2 out]
              }
              frame "p" {
                n698 = Generate User Event "action User Event"(user event=w1380, event data cluster="action: copy to math" ("event data")) -> ()  [unwired: 2 in, 2 out]
              }
              frame "q" {
                n699 = Generate User Event "action User Event"(user event=w1382, event data cluster="action: copy from math" ("event data")) -> ()  [unwired: 2 in, 2 out]
              }
              frame "\\", "|" {
                n700 = for {
                  N: 1 -> [_]
                  tunnel: w1386 -> [w1400]
                  tunnel: w1384 -> [w1399]
                  tunnel: [w1399] -> w1383
                  n701 = property on="selection :|\\" class="Ring (strict)"() -> ("NumItems"=w1389:u32)  [unwired: 2 in, 2 out]
                  n702 = local read "selection :|\\"() -> (w1391:u16)
                  n703 = To Long Integer(number=w1391) -> (32bit integer=w1390:i32)
                  n704 = case shown="\"|\", Default" w1400 {
                    tunnel: w1390 -> [w1402 w1404]
                    tunnel: [w1401 w1403] -> w1396
                    frame "|", Default {
                      n705 = Decrement(x=w1402) -> (x-1=w1401:i32)
                    }
                    frame "\\" {
                      n706 = Increment(x=w1404) -> (x+1=w1403:i32)
                    }
                  }
                  n707 = To Long Integer(number=w1389) -> (32bit integer=w1388:i32)
                  n708 = Greater Or Equal?(x=w1396, y=w1388) -> (x >= y?=w1398:bool)
                  n709 = Select(t=u16 0 ("lower limit"), s=w1398, f=w1396) -> (s? t:f=w1393:i32)
                  n710 = Decrement(x=w1388) -> (x-1=w1394:i32)
                  n711 = Less Than 0?(x=w1393) -> (x < 0?=w1395:bool)
                  n712 = Select(t=w1394, s=w1395, f=w1393) -> (s? t:f=w1392:i32)
                  n713 = local write "selection :|\\"(w1392) -> ()
                }
                n714 = Generate User Event ("action User Event")(user event=w1383, event data cluster="action: constrained filenames select" ("event data")) -> ()  [unwired: 2 in, 2 out]
              }
              frame "m" {
                n715 = Generate User Event "action User Event"(user event=w1405, event data cluster="action: copy from math" ("event data")) -> ()  [unwired: 2 in, 2 out]
              }
            }
          }
          frame "Escape" {
            n716 = local write "newton pause"(TRUE ("newton pause")) -> ()
          }
          frame "PageUp" {
          }
          frame "Enter" {
            n717 = Generate User Event ("action User Event")(user event=w1408, event data cluster="action: new sweep" ("event data")) -> (user event out=w1409:refnum<user-event>)  [unwired: 2 in, 1 out]
            n718 = Generate User Event ("action User Event")(user event=w1409, event data cluster="action: replot colors" ("event data")) -> ()  [unwired: 2 in, 2 out]
          }
          frame "Caps" {
          }
          frame "PageDown" {
          }
          frame "Up".."Right" {
            n719 = case shown="\"Down\"" w1413 {
              tunnel: [cursor_action."zoom in 20%" ("cursor action") cursor_action."zoom out 20%" ("cursor action") cursor_action."zoom out 20%" ("cursor action") cursor_action."zoom in 20%" ("cursor action")] -> w1414
